vi "Counts.vi"() -> ()   [LabVIEW 2011]
doc: "This sample project is built upon the standard state machine template and shows how you could create an application that acquires, analyzes, and presents data. It includes functionality for presenting configuration dialogs, preserving settings between executions, loading and saving data, as well as exporting graph images and text files.\n\nIt is most appropriate for data that is acquired instantly as it does not allow for screen updates mid acquisition nor does it allow for continuous streaming to disk."
panel:
  in  "Runs":dbl=100.0
  in  "Pulse TTL 2":bool
  in  "Pulse TTL 1":bool
  in  "Toggle\nTTL 2":bool
  in  "Toggle\nTTL 1":bool
  in  "Record\nstatistics":bool
  in  "Raw Data\nFile Name 2":string="C:\\FPGA\\stats.txt"
  in  "Clock Freq. [MHz]":dbl=48.0
  in  "Record\nraw data":bool
  out "Elapsed time (s)":dbl
  out "FPGA Counts\nStatus":dbl
  out "USB Open\nStatus":dbl
  out "Channel 4 Total\nCounts":dbl
  out "Channel 3 Total\nCounts":dbl
  out "Channel 2 Total\nCounts":dbl
  out "Channel 1 Total\nCounts":dbl
  in  "Raw Data\nFile Name":string="C:\\FPGA\\raw.txt"
  out "?":dbl
  out "?":dbl
  out "?":dbl
  out "?":dbl
  out "stats":i64[](array[numeric])
  in  "Stop":bool
  out "Channel 4 CPS":dbl(knob) scale=0.0..1000000.0
  out "Channel 3 CPS":dbl(knob) scale=0.0..1000000.0
  out "Channel 2 CPS":dbl(knob) scale=0.0..1000000.0
  out "Channel 1 CPS":dbl(knob) scale=0.0..1000000.0
  # "Clocks"
  # "Channel 1"
  # "Channel 2"
  # "Channel 3"
  # "Channel 4"
  # "Coincidence Channels 1 & 2"
  # "Coincidence Channels 1 & 3"
  # "Coincidence Channels 1 & 4"
  # "Coincidence Channels 2 & 3"
  # "Coincidence Channels 2 & 4"
  # "Coincidence Channels 3 & 4"
  # "Coincidence Channels 1 & 2 & 3"
  # "Coincidence Channels 1 & 2 & 4"
  # "Coincidence Channels 1 & 3 & 4"
  # "Coincidence Channels 2 & 3 & 4"
  # "Coincidence Channels 1 & 2 & 3 & 4"
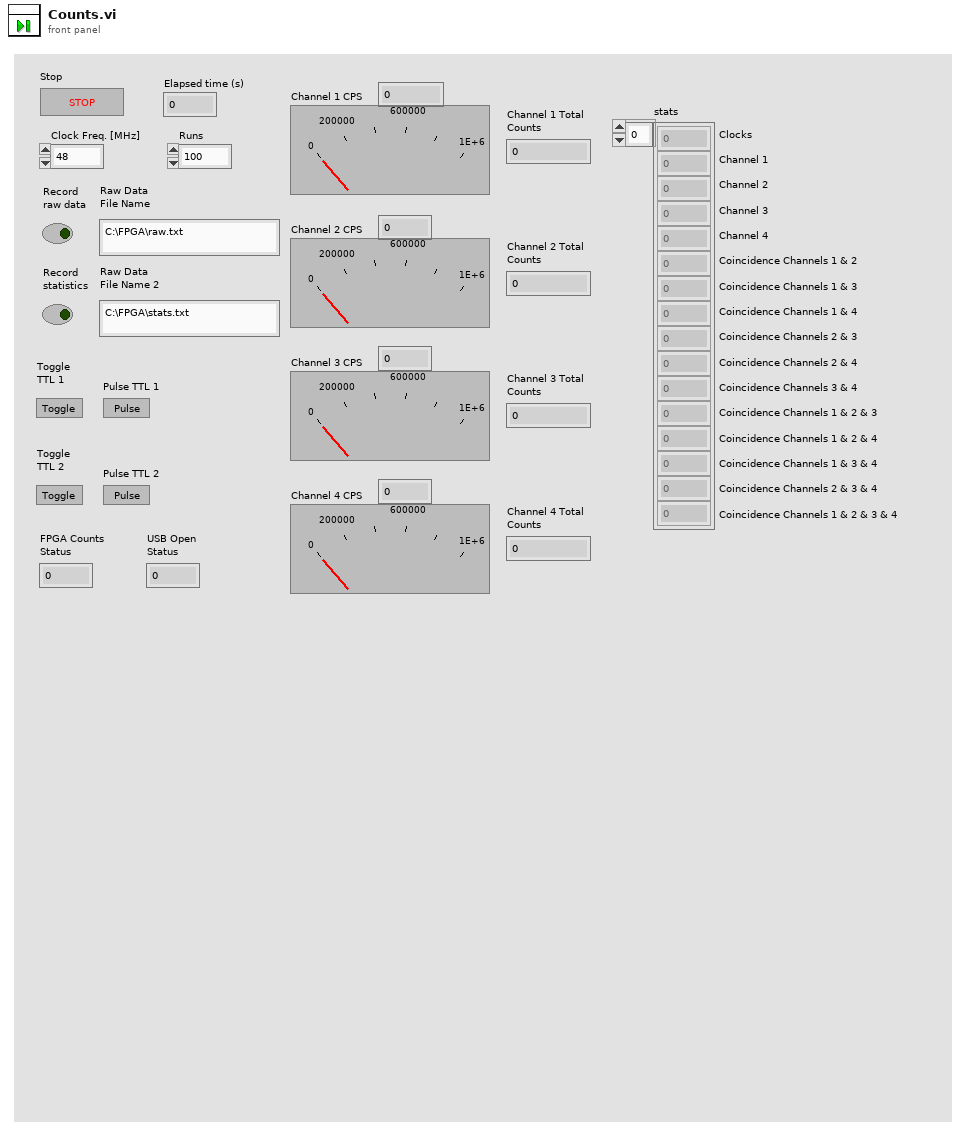
[diagram p1: front panel]
types:
  T1 = enum16{"open", "replace", "create", "open or create", "replace or create", "replace or create with confirmation"}
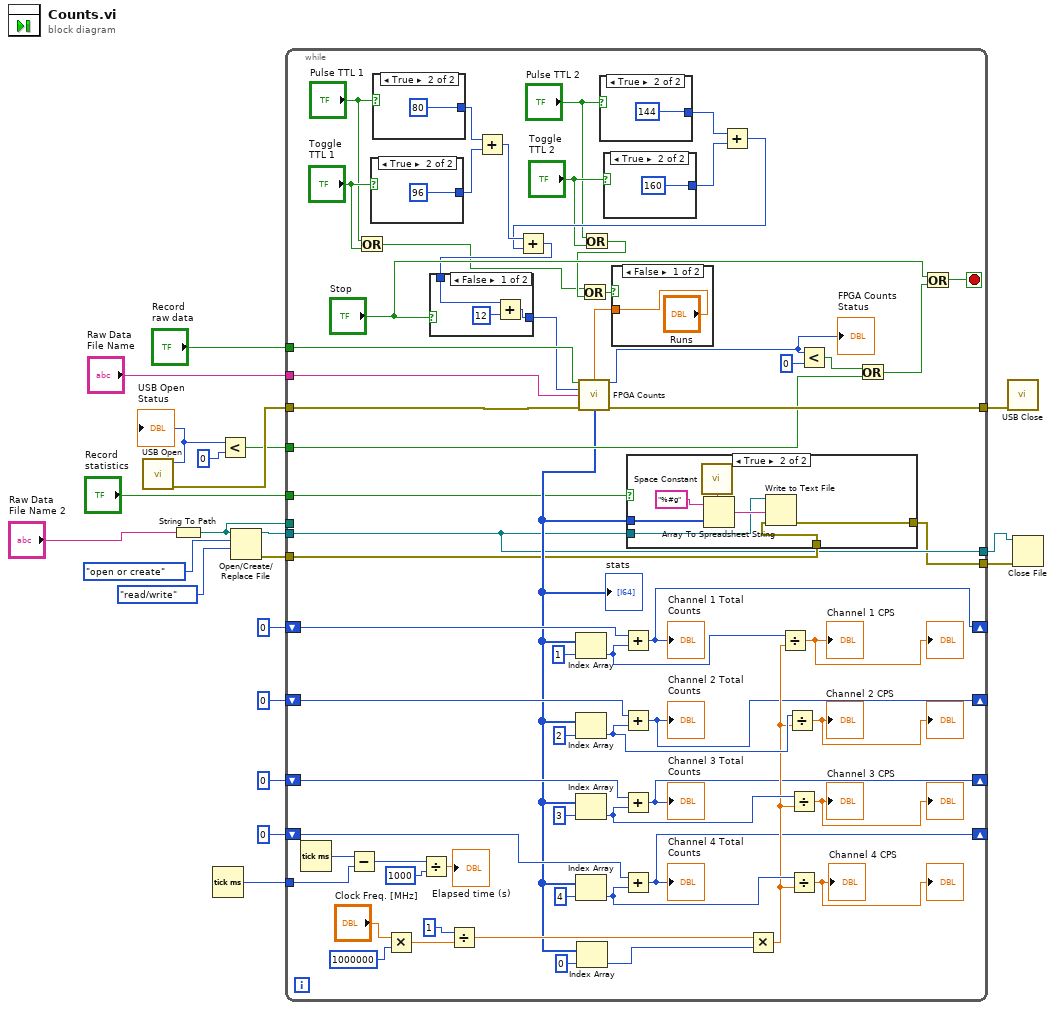
[diagram p0: block diagram]
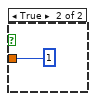
[diagram p2: hidden frame]
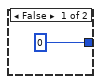
[diagram p3: hidden frame]
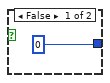
[diagram p4: hidden frame]
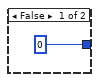
[diagram p5: hidden frame]
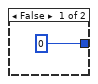
[diagram p6: hidden frame]
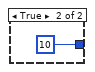
[diagram p8: hidden frame]
diagram:
  n1 = call "USB Open.vi"() -> ("error out"=w15:errorcluster, "function return"=w12:i32)  [unwired: 10 in]
  "USB Open\nStatus" <- w12
  n2 = String To Path(string="Raw Data\nFile Name 2") -> (path=w4:path)
  n3 = Tick Count (ms)() -> (millisecond timer value=w10:u32)
  n4 = Less?(x=w12, y=0) -> (x < y?=w11:bool)
  n5 = Open/Create/Replace File(file path (use dialog)=w4, operation (0:open)=T1."open or create", access (0:read/write)=enum16{"read/write", "read-only", "write-only"}."read/write") -> (refnum out=w3:refnum<file>, error out=w5:errorcluster)  [unwired: 3 in, 1 out]
  n6 = while {
    shift-right: [w47] -> _
    shift-left: 0 -> [w77]
    shift-right: [w46] -> _
    shift-left: 0 -> [w78]
    shift-right: [w45] -> _
    shift-left: 0 -> [w79]
    shift-right: [w44] -> _
    shift-left: 0 -> [w80]
    tunnel: w15 -> [w22]
    tunnel: [w55] -> w14
    tunnel: "Record\nraw data" -> [w57]
    tunnel: "Raw Data\nFile Name" -> [w54]
    tunnel: w11 -> [w51]
    tunnel: w10 -> [w43]
    tunnel: "Record\nstatistics" -> [w40]
    tunnel: w5 -> [w39]
    tunnel: w4 -> [_]
    tunnel: w3 -> [w38]
    tunnel: [w38] -> w2
    tunnel: [w37] -> w1
    stop <- w48 stop-if-true
    n7 = Tick Count (ms)() -> (millisecond timer value=w66:u32)
    n8 = Subtract(x=w66, y=w43) -> (x-y=w86:u32)
    n9 = Or(x="Pulse TTL 1", y="Toggle\nTTL 1") -> (x .or. y?=w23:bool)
    n10 = case shown="True" "Toggle\nTTL 1" {
      tunnel: [0 96] -> w35
      frame False {
      }
      frame True {
      }
    }
    n11 = case shown="True" "Pulse TTL 1" {
      tunnel: [0 80] -> w36
      frame False {
      }
      frame True {
      }
    }
    n12 = Multiply(x="Clock Freq. [MHz]", y=1000000) -> (x*y=w64:dbl)
    n13 = Divide(x=w86, y=1000) -> (x/y=→"Elapsed time (s)":dbl)
    n14 = Divide(x=1, y=w64) -> (x/y=w62:dbl)
    n15 = Add(x=w36, y=w35) -> (x+y=w34:i32)
    n16 = Or(x="Pulse TTL 2", y="Toggle\nTTL 2") -> (x .or. y?=w28:bool)
    n17 = Or(x=w23, y=w28) -> (x .or. y?=w29:bool)
    n18 = case shown="True" "Pulse TTL 2" {
      tunnel: [0 144] -> w31
      frame False {
      }
      frame True {
      }
    }
    n19 = case shown="True" "Toggle\nTTL 2" {
      tunnel: [0 160] -> w32
      frame False {
      }
      frame True {
      }
    }
    n20 = case shown="False" w29 {
      tunnel: ["Runs" 1] -> w56
      frame False {
      }
      frame True {
      }
    }
    n21 = Add(x=w31, y=w32) -> (x+y=w30:i32)
    n22 = Add(x=w34, y=w30) -> (x+y=w33:i32)
    n23 = case shown="False" "Stop" {
      tunnel: [w106 10] -> w52
      tunnel: w33 -> [w105 _]
      frame False {
        n24 = Add(x=w105, y=12) -> (x+y=w106:i32)
      }
      frame True {
      }
    }
    n25 = call "FPGA Counts.vi"("saveData"=w57, "runs"=w56, "fpgaCommand"=w52, "fileName"=w54, "error in (no error)"=w22) -> ("function return"=w53:i32, "stats"=w41:i64[], "error out"=w55:errorcluster)  [unwired: 6 in, 2 out]
    "stats" <- w41
    "FPGA Counts\nStatus" <- w53
    n26 = Index Array(array=w41, index=1) -> (element=w70:i64)
    n27 = Index Array(array=w41, index=2) -> (element=w69:i64)
    n28 = Index Array(array=w41, index=3) -> (element=w68:i64)
    n29 = Index Array(array=w41, index=4) -> (element=w67:i64)
    n30 = Index Array(array=w41, index=0) -> (element=w60:i64)
    n31 = Add(x=w77, y=w70) -> (x+y=w47:i64)
    "Channel 1 Total\nCounts" <- w47
    n32 = Add(x=w78, y=w69) -> (x+y=w46:i64)
    "Channel 2 Total\nCounts" <- w46
    n33 = Add(x=w79, y=w68) -> (x+y=w45:i64)
    "Channel 3 Total\nCounts" <- w45
    n34 = Add(x=w80, y=w67) -> (x+y=w44:i64)
    "Channel 4 Total\nCounts" <- w44
    n35 = case shown="True" w40 {
      tunnel: w41 -> [_ w102]
      tunnel: w39 -> [w97 w99]
      tunnel: w38 -> [_ w100]
      tunnel: [w97 w98] -> w37
      frame False {
      }
      frame True {
        n36 = call <vilib>:"Space Constant.vi"() -> ("String"=w104:string)
        n37 = Array To Spreadsheet String(delimiter (Tab)=w104, array=w102, 3:"%#g") -> (spreadsheet string=w101:string)
        n38 = Write to Text File(file (use dialog)=w100, text=w101, error in=w99) -> (error out=w98:errorcluster)  [unwired: 1 in, 2 out]
      }
    }
    n39 = Multiply(x=w62, y=w60) -> (x*y=w65:dbl)
    n40 = Divide(x=w70, y=w65) -> (x/y=→"Channel 1 CPS" →"?":dbl)
    n41 = Divide(x=w69, y=w65) -> (x/y=→"Channel 2 CPS" →"?":dbl)
    n42 = Divide(x=w68, y=w65) -> (x/y=→"Channel 3 CPS" →"?":dbl)
    n43 = Divide(x=w67, y=w65) -> (x/y=→"Channel 4 CPS" →"?":dbl)
    n44 = Less?(x=w53, y=0) -> (x < y?=w50:bool)
    n45 = Or(x=w50, y=w51) -> (x .or. y?=w49:bool)
    n46 = Or(x="Stop", y=w49) -> (x .or. y?=w48:bool)
  }
  n47 = call "USB Close.vi"("error in (no error)"=w14) -> ()  [unwired: 9 in, 2 out]
  n48 = Close File(refnum=w2, error in=w1) -> ()  [unwired: 2 out]
